vi "String.Multiple Text Control Input Check.vi"(11 "Array":refnum<vi>[](array[refnum])) -> (2 "NextFocus":i32, 3 "AllFilled":bool)   [LabVIEW 2019]
panel:
  in  "Test":bool
  in  "String 3":string
  in  "String 2":string
  in  "String":string
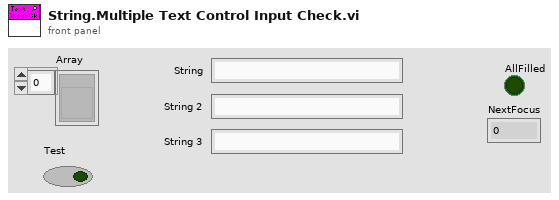
[diagram p1: front panel]
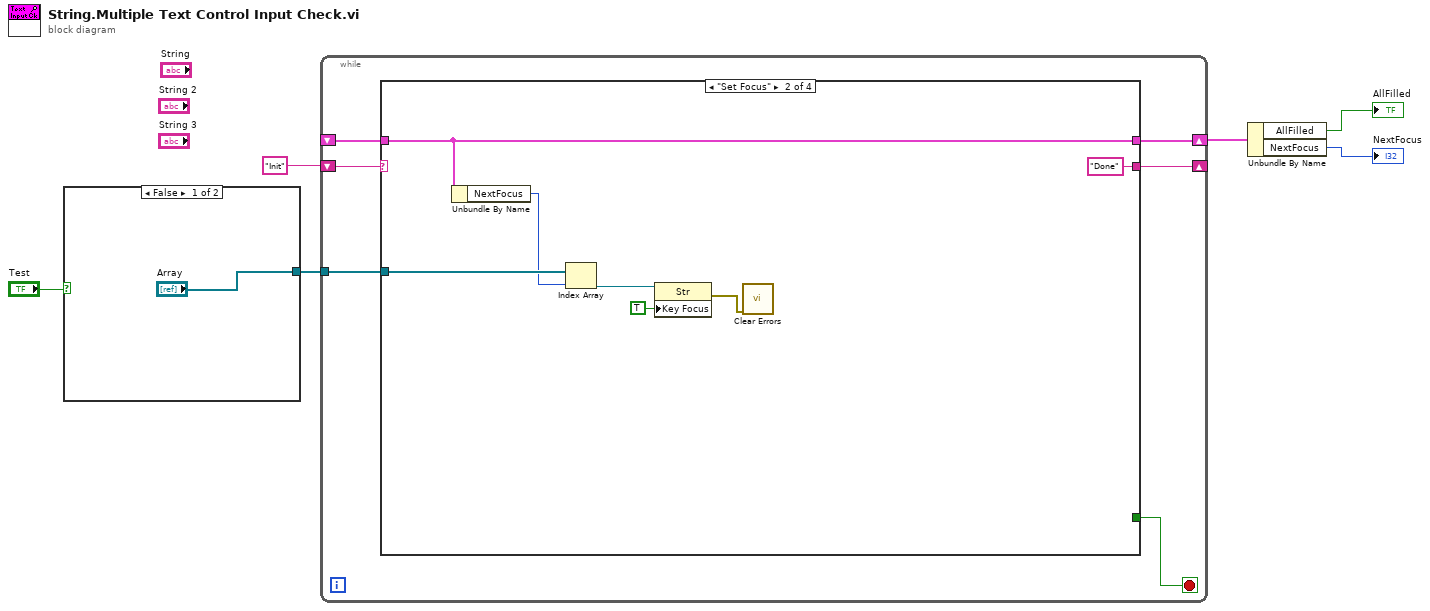
[diagram p0: block diagram]
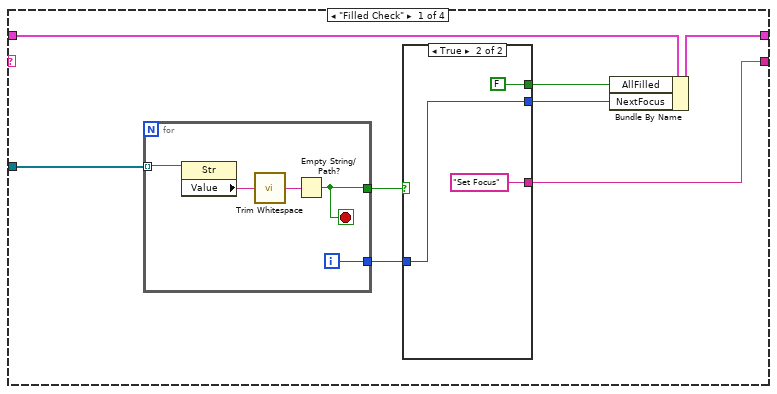
[diagram p2: hidden frame]
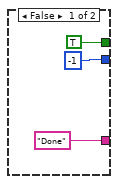
[diagram p3: hidden frame]
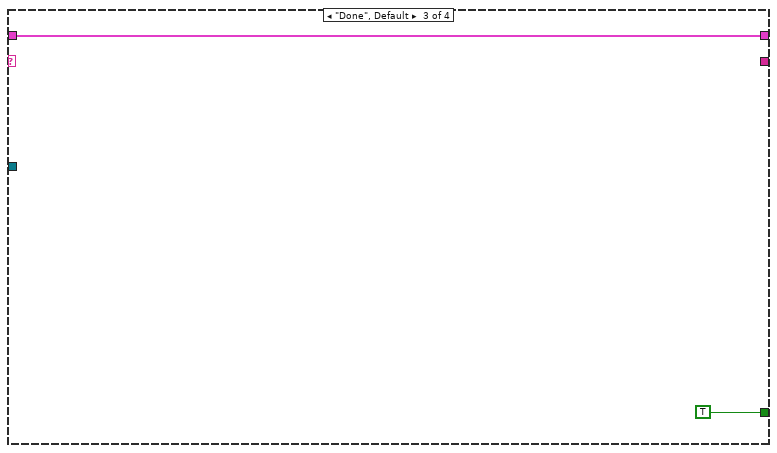
[diagram p4: hidden frame]
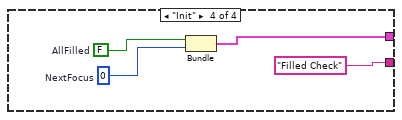
[diagram p5: hidden frame]
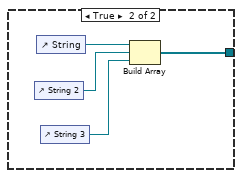
[diagram p6: hidden frame]
diagram:
  n1 = case shown="False" "Test" {
    tunnel: ["Array" w8] -> w5
    frame False {
    }
    frame True {
      n2 = control-ref of="String 2"() -> (w10:refnum<vi>)
      n3 = control-ref of="String"() -> (w11:refnum<vi>)
      n4 = control-ref of="String 3"() -> (w9:refnum<vi>)
      n5 = Build Array(w11, w10, w9) -> (w8:refnum<vi>[])
    }
  }
  n6 = while {
    tunnel: w5 -> [w13]
    shift-right: [w14] -> _
    shift-left: "Init" -> [w17]
    shift-right: [w15] -> w3
    shift-left: _ -> [w16]
    stop <- w12 stop-if-true
    n7 = case shown="\"Set Focus\"" w17 {
      tunnel: w16 -> [w23 w41 w44 _]
      tunnel: [w24 w41 w44 w47] -> w15
      tunnel: [w18 "Done" _ "Filled Check"] -> w14
      tunnel: w13 -> [w25 w43 _ _]
      tunnel: [_ _ TRUE _] -> w12
      frame "Filled Check" {
        n8 = for {
          tunnel: w25 -> [w36] mode=indexing
          tunnel: [w35] -> w21
          tunnel: [w32] -> w22
          i -> [w35]
          stop <- w32 stop-if-true
          n9 = property class="Str"(reference=w36) -> ("Value"=w33:string)  [unwired: 1 in, 2 out]
          n10 = call <vilib>:"Trim Whitespace.vi"("string"=w33) -> ("trimmed string"=w34:string)  [unwired: 1 in]
          n11 = Empty String/Path?(string/path=w34) -> (empty?=w32:bool)
        }
        n12 = case shown="True" w22 {
          tunnel: w21 -> [_ w31]
          tunnel: [-1 w31] -> w20
          tunnel: [TRUE FALSE] -> w19
          tunnel: ["Done" "Set Focus"] -> w18
          frame False {
          }
          frame True {
          }
        }
        n13 = Bundle By Name(cluster=w23, "AllFilled"=w19, "NextFocus"=w20) -> (w24:cluster{"AllFilled":bool, "NextFocus":i32})
      }
      frame "Set Focus" {
        n14 = Unbundle By Name(w41) -> ("NextFocus"=w40:i32)
        n15 = Index Array(array=w43, index=w40) -> (element=w42:refnum<vi>)
        n16 = property class="Str"(reference=w42, "Key Focus"=TRUE) -> (error out=w38:errorcluster)  [unwired: 1 in, 1 out]
        n17 = call <vilib>:"Clear Errors.vi"("error in (no error)"=w38) -> ()  [unwired: 5 in, 2 out]
      }
      frame "Done", Default {
      }
      frame "Init" {
        w48 = 0  # NextFocus
        w49 = FALSE  # AllFilled
        n18 = Bundle("AllFilled"=w49, "NextFocus"=w48) -> (w47:cluster{"AllFilled":bool, "NextFocus":i32})  [unwired: 1 in]
      }
    }
  }
  n19 = Unbundle By Name(w3) -> ("AllFilled"=→"AllFilled":bool, "NextFocus"=→"NextFocus":i32)
